vi "4155C DOWNLOAD variable.vi"(4 "error in (no error)":errorcluster, 6 "Variable name":string, 7 "VISA resource name in":refnum<visa-resource-name>) -> (0 "error out":errorcluster, 2 "Output data":dbl[](array[numeric]) format="%.2f", 3 "VISA Resource Name out":refnum<visa-resource-name>)   [LabVIEW 2019]
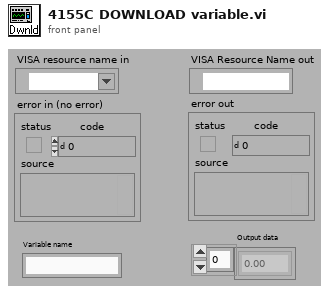
[diagram p1: front panel]
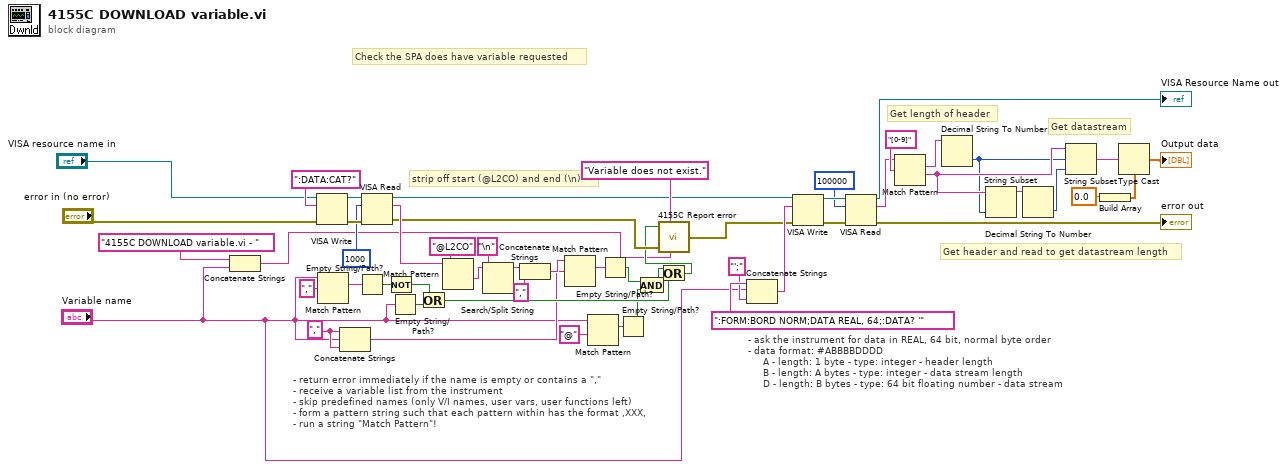
[diagram p0: block diagram]
diagram:
  w43 = ","
  # "Get datastream"
  # "Get header and read to get datastream length"
  # "Get length of header"
  # "Check the SPA does have variable requested"
  # "- ask the instrument for data in REAL, 64 bit, normal byte order\n- data format: #ABBBBDDDD \n     A - length: 1 byte - type: integer - header length\n     B - length: A bytes - type: integer - data stream length\n     D - length: B bytes - type: 64 bit floating number - data stream"
  # "strip off start (@L2CO) and end (\\n)"
  # "- return error immediately if the name is empty or contains a \",\"\n- receive a variable list from the instrument\n- skip predefined names (only V/I names, user vars, user functions left)\n- form a pattern string such that each pattern within has the format ,XXX,\n- run a string \"Match Pattern\"!"
  n1 = Concatenate Strings("4155C DOWNLOAD variable.vi - " ("Substring"), "Variable name") -> (w28:string)
  n2 = VISA Write(VISA resource name="VISA resource name in", write buffer=":DATA:CAT?", error in (no error)="error in (no error)") -> (VISA resource name out=w50:refnum<visa-resource-name>, error out=w49:errorcluster)  [unwired: 1 out]
  n3 = Match Pattern(string="Variable name", regular expression=",") -> (match substring=w52:string)  [unwired: 1 in, 3 out]
  n4 = Concatenate Strings(w43, "Variable name", w43) -> (w32:string)
  n5 = Empty String/Path?(string/path=w52) -> (empty?=w51:bool)
  n6 = VISA Read(VISA resource name=w50, byte count=1000, error in (no error)=w49) -> (VISA resource name out=w10:refnum<visa-resource-name>, read buffer=w47:string, error out=w35:errorcluster)  [unwired: 1 out]
  n7 = Not(x=w51) -> (.not. x?=w45:bool)
  n8 = Empty String/Path?(string/path="Variable name") -> (empty?=w44:bool)
  n9 = Or(x=w45, y=w44) -> (x .or. y?=w37:bool)
  n10 = Match Pattern(string=w47, regular expression="@L2CO") -> (after substring=w42:string)  [unwired: 1 in, 3 out]
  n11 = Search/Split String(string=w42, search string/char (-)="\n") -> (substring before match=w40:string)  [unwired: 1 in, 2 out]
  n12 = Concatenate Strings(w40, ",") -> (w38:string)
  n13 = Match Pattern(string=w38, regular expression=w32) -> (match substring=w36:string)  [unwired: 1 in, 3 out]
  n14 = Match Pattern(string="Variable name", regular expression="@") -> (match substring=w4:string)  [unwired: 1 in, 3 out]
  n15 = Empty String/Path?(string/path=w36) -> (empty?=w3:bool)
  n16 = Empty String/Path?(string/path=w4) -> (empty?=w1:bool)
  n17 = And(x=w3, y=w1) -> (x .and. y?=w2:bool)
  n18 = Or(x=w37, y=w2) -> (x .or. y?=w33:bool)
  n19 = call "4155C Report error.vi"("new error"=w33, "error message"="Variable does not exist.", "error in (no error)"=w35, "source"=w28) -> ("error out"=w11:errorcluster)  [unwired: 1 in]
  n20 = Concatenate Strings(":FORM:BORD NORM;DATA REAL, 64;:DATA? '", "Variable name", "';") -> (w23:string)
  n21 = VISA Write(VISA resource name=w10, write buffer=w23, error in (no error)=w11) -> (VISA resource name out=w27:refnum<visa-resource-name>, error out=w26:errorcluster)  [unwired: 1 out]
  n22 = VISA Read(VISA resource name=w27, byte count=100000, error in (no error)=w26) -> (VISA resource name out=→"VISA Resource Name out":refnum<visa-resource-name>, read buffer=w12:string, error out=→"error out":errorcluster)  [unwired: 1 out]
  n23 = Match Pattern(string=w12, regular expression="[0-9]") -> (match substring=w21:string, after substring=w19:string)  [unwired: 1 in, 2 out]
  n24 = Decimal String To Number(string=w21) -> (number=w18:i32)  [unwired: 2 in, 1 out]
  n25 = String Subset(string=w19, length (rest)=w18) -> (substring=w17:string)  [unwired: 1 in]
  n26 = Decimal String To Number(string=w17) -> (number=w16:i32)  [unwired: 2 in, 1 out]
  n27 = String Subset(string=w19, offset (0)=w18, length (rest)=w16) -> (substring=w14:string)
  n28 = Build Array(0.0) -> (w15:dbl[])
  n29 = Type Cast(type=w15, x=w14) -> (*(type *) &x=→"Output data":dbl[])
